vi "Find Areas That Can Contain a Beacon.vi"(0 "Sensors":map{T2, T3}(c390), 1 "Boundary":T1={"X Max"=4000000, "X Min"=0, "Y Max"=4000000, "Y Min"=0}) -> (2 "Area Centroids":cluster{"Centroid X":dbl, "Centroid Y":dbl}[](array[cluster]) {"Centroid X" format="%#_15f"; "Centroid Y" format="%#_15f"}, 3 "Area That Can Contain Beacons":cluster{cluster{"X":dbl, "Y":dbl}[]}[](graph))   [LabVIEW 2020, in "AoC 2022.lvlib"]
uses:
  AoC 2022.lvlib
  Location.ctl
  Sensor Info.ctl
  Coverage Area.ctl
  <vilib>/4SmartMachines/Polygon Clipping/polyClipping.lvlib
  <vilib>/Analysis/NI_AAL_Geometry.lvlib
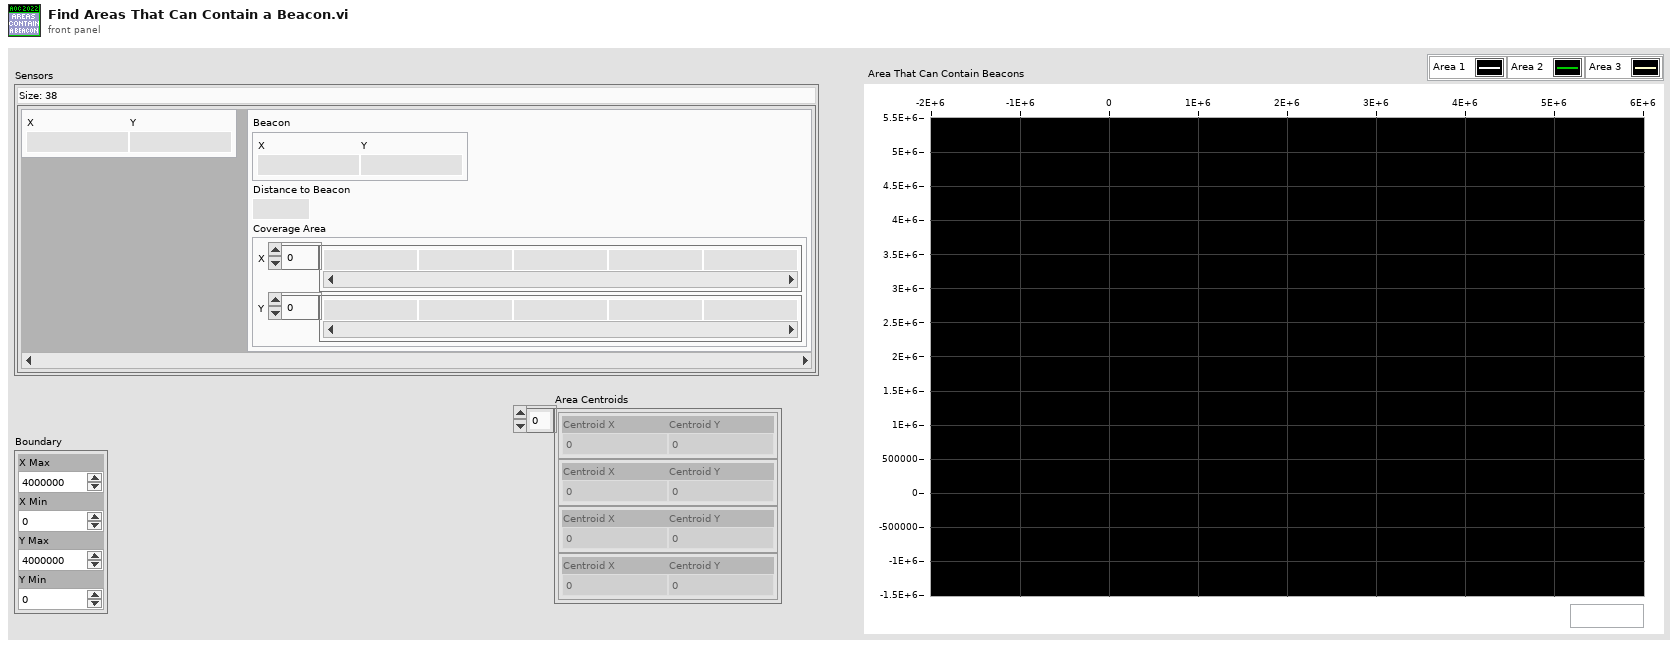
[diagram p1: front panel]
types:
  T1 = cluster{"X Max":i32, "X Min":i32, "Y Max":i32, "Y Min":i32}
  T2 = typedef "AoC 2022.lvlib/Location.ctl" = cluster{"X":i32, "Y":i32}
  T3 = typedef "AoC 2022.lvlib/Sensor Info.ctl" = cluster{"Beacon":T2, "Distance to Beacon":dbl, "Coverage Area":T4}
  T4 = typedef "AoC 2022.lvlib/Coverage Area.ctl" = cluster{"X":dbl[], "Y":dbl[]}
  T5 = enum16{"Intersection", "Union", "Difference", "Xor"}
  T6 = cluster{"X Max":dbl, "X Min":dbl, "Y Max":dbl, "Y Min":dbl}
  T7 = cluster{"Points":cluster{"X":dbl, "Y":dbl}[], "Hole":bool}[]
  T8 = cluster{cluster{"X Max":dbl, "Y Min":dbl}[], bool}
  T9 = cluster{cluster{"X Max":dbl, "Y Min":dbl}[], bool}[]
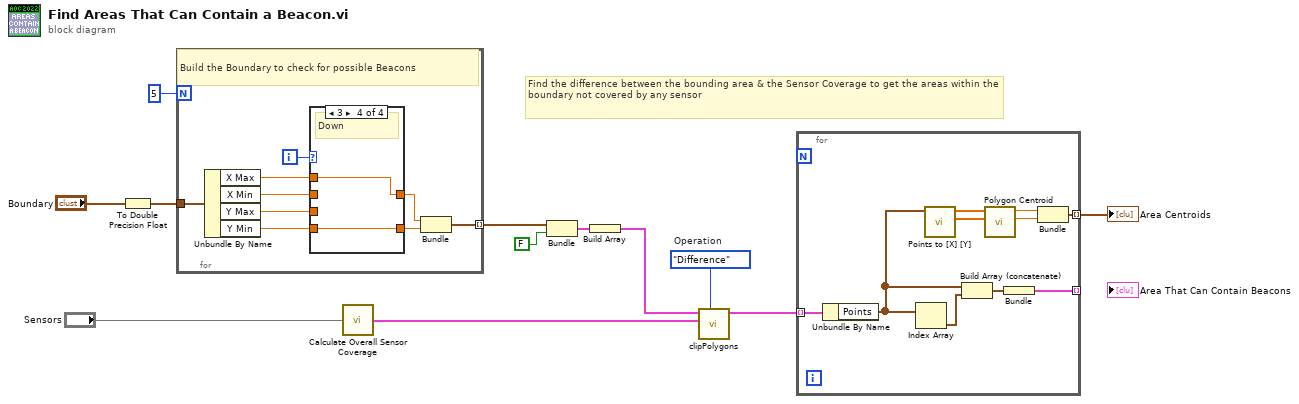
[diagram p0: block diagram]
diagram:
  w11 = T5."Difference"  # Operation
  # "Find the difference between the bounding area & the Sensor Coverage to get the areas within the boundary not covered by any sensor"
  n1 = To Double Precision Float(number="Boundary") -> (double precision float=w8:T6)
  n2 = for {
    N: 5 -> [_]
    tunnel: w8 -> [w20]
    tunnel: [w15] -> w7 mode=indexing
    i -> [w21]
    # "Build the Boundary to check for possible Beacons"
    n3 = Unbundle By Name(w20) -> ("X Max"=w19:dbl, "X Min"=w18:dbl, "Y Max"=w17:dbl, "Y Min"=w16:dbl)
    n4 = case shown="3" w21 {
      tunnel: w19 -> [_ _ w26 w29]
      tunnel: w18 -> [w23 w25 _ _]
      tunnel: w17 -> [_ w24 w27 _]
      tunnel: w16 -> [w22 _ _ w28]
      tunnel: [w23 w25 w26 w29] -> w14
      tunnel: [w22 w24 w27 w28] -> w13
      frame 0, 4, Default {
        # "Left"
      }
      frame 1 {
        # "Top"
      }
      frame 2 {
        # "Right"
      }
      frame 3 {
        # "Down"
      }
    }
    n5 = Bundle("X Max"=w14, "Y Min"=w13) -> (w15:cluster{"X Max":dbl, "Y Min":dbl})  [unwired: 1 in]
  }
  n6 = call "Calculate Overall Sensor Coverage.vi"("Sensors"="Sensors") -> ("Overall Sensor Coverage"=w2:T7)
  n7 = Bundle(w7, FALSE) -> (w5:T8)  [unwired: 1 in]
  n8 = Build Array(w5) -> (w4:T9)
  n9 = call <vilib>:"clipPolygons.vi"("Operation"=w11, "Polygon Set 2"=w2, "Polygon Set 1"=w4) -> ("Polygon Set Out"=w12:T7)  [unwired: 7 in, 1 out]
  n10 = for {
    tunnel: w12 -> [w39] mode=indexing
    tunnel: [w38] -> _ mode=indexing
    tunnel: [w30] -> w3 mode=indexing
    n11 = Unbundle By Name(w39) -> ("Points"=w35:cluster{"X":dbl, "Y":dbl}[])
    n12 = Index Array(array=w35) -> (element=w37:cluster{"X":dbl, "Y":dbl})  [unwired: 1 in]
    n13 = call "Points to [X] [Y].vi"("Points"=w35) -> ("Y"=w33:dbl[], "X"=w34:dbl[])  [unwired: 9 in]
    n14 = Build Array (concatenate)(w35, w37) -> (w36:cluster{"X":dbl, "Y":dbl}[])
    n15 = call <vilib>:"Polygon Centroid.vi"("Y"=w33, "X"=w34) -> ("Centroid Y"=w31:dbl, "Centroid X"=w32:dbl)  [unwired: 7 in, 1 out]
    n16 = Bundle(w36) -> (w38:cluster{cluster{"X":dbl, "Y":dbl}[]})  [unwired: 1 in]
    n17 = Bundle("Centroid X"=w32, "Centroid Y"=w31) -> (w30:cluster{"Centroid X":dbl, "Centroid Y":dbl})  [unwired: 1 in]
  }
  "Area Centroids" <- w3
